vi "Close Module.vi"(7 "Self":refnum<class "UniqueName.lvclass">, 8 "error in (no error)":errorcluster, 9 "Wait for stop?":bool, 11 "Module Admin in":refnum<class "Delacor_lib_QMH_Cloneable Module Admin.lvclass">) -> (0 "error out":errorcluster, 1 "External Launch":bool, 3 "Module Admin out":refnum<class "Delacor_lib_QMH_Cloneable Module Admin.lvclass">)   [LabVIEW 2014, in "Configurable.lvlib"]
doc: "Destroy the Broadcast Events and Request Events (if this was the first instance). Reset flags stored in Module Admin class.\n_____\nBased on Delacor QMH Project Template 4.0.0.47."
uses:
  Configurable.lvlib
  <vilib>/Delacor/Delacor QMH/Libraries/Cloneable Module Admin_class/Delacor_lib_QMH_Cloneable Module Admin.lvclass
  <vilib>/LabVIEW Open Source Project/Unicity/UniqueName/UniqueNameClass/UniqueName.lvclass
  <vilib>/Delacor/Delacor QMH/Libraries/Cloneable Module Admin_class/Delacor_lib_QMH_Cloneable Module Admin.lvclass/Delacor_lib_QMH_Cloneable Module Admin.ctl
  <vilib>/Delacor/Delacor QMH/Libraries/Module Admin_class/Delacor_lib_QMH_Module Admin.lvclass/Delacor_lib_QMH_Module Admin.ctl
  <vilib>/Delacor/Delacor QMH/Libraries/Cloneable Module Admin_class/Delacor_lib_QMH_Get First.vi
  <vilib>/Delacor/Delacor QMH/Libraries/Cloneable Module Admin_class/Delacor_lib_QMH_Get Module ID.vi
  <vilib>/Delacor/Delacor QMH/Libraries/Module Admin_class/Delacor_lib_QMH_Get External Launch.vi
  Clone Registration/Clone Registration.lvlib
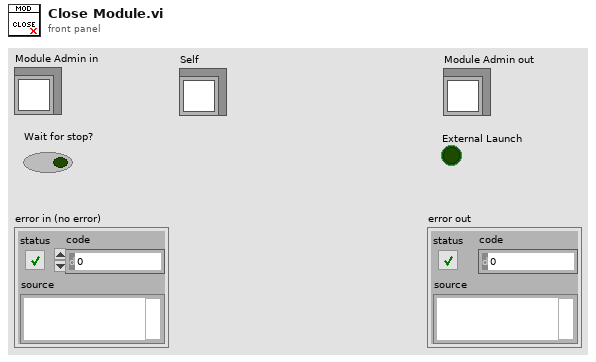
[diagram p1: front panel]
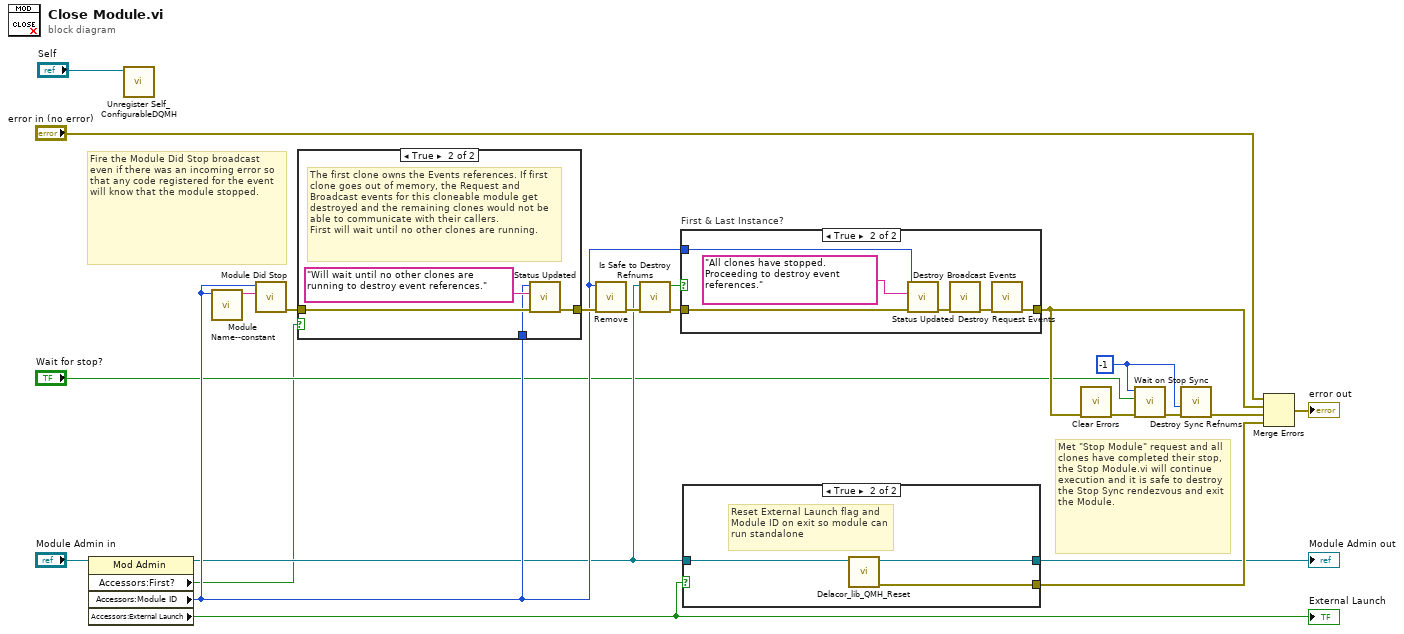
[diagram p0: block diagram]
diagram:
  w8 = -1 ("Module ID")
  # "Fire the Module Did Stop broadcast even if there was an incoming error so that any code registered for the event will know that the module stopped."
  # "Met \"Stop Module\" request and all clones have completed their stop, the Stop Module.vi will continue execution and it is safe to destroy the Stop Sync rendezvous and exit the Module."
  n1 = property class="Mod Admin"(reference="Module Admin in") -> (reference out=w17:refnum<class "Delacor_lib_QMH_Cloneable Module Admin.lvclass">, "Accessors:First?"=w5:bool, "Accessors:Module ID"=w21:i32, "Accessors:External Launch"=w4:bool)  [unwired: 1 in, 1 out]
  "External Launch" <- w4
  n2 = call "Unregister Self_ConfigurableDQMH.vi"("Self"="Self") -> ()  [unwired: 11 in]
  n3 = call "Module Name--constant.vi"("Module ID"=w21) -> ("Module Name"=w3:string)  [unwired: 10 in]
  n4 = call "Module Did Stop.vi"("Origin"=w3, "Module ID"=w21) -> ("error out"=w12:errorcluster)  [unwired: 9 in]
  n5 = case shown="True" w5 {
    tunnel: w12 -> [w23 w27]
    tunnel: w21 -> [_ w25]
    tunnel: [w23 w24] -> w22
    frame False {
    }
    frame True {
      # "The first clone owns the Events references. If first clone goes out of memory, the Request and Broadcast events for this cloneable module get destroyed and the remaining clones would not be able to communicate with their callers.\nFirst will wait until no other clones are running."
      n6 = call "Status Updated.vi"("error in (no error)"=w27, "Status"="Will wait until no other clones are running to destroy event references." ("format string"), "Module ID"=w25) -> ("error out"=w24:errorcluster)  [unwired: 8 in]
    }
  }
  n7 = call "Remove.vi"("error in (no error)"=w22, "Module ID"=w21) -> ("error out"=w18:errorcluster)  [unwired: 8 in, 1 out]
  n8 = call "Is Safe to Destroy Refnums.vi"("error in (no error)"=w18, "Module Admin"=w17) -> ("error out"=w14:errorcluster, "Destroy Broadcast & Request Event Refs?"=w15:bool)  [unwired: 8 in]
  n9 = case "First & Last Instance?" shown="True" w15 {
    tunnel: w14 -> [w28 w32]
    tunnel: [w28 w34] -> w20
    tunnel: w21 -> [_ w30]
    frame False {
    }
    frame True {
      n10 = call "Status Updated.vi"("error in (no error)"=w32, "Status"="All clones have stopped. Proceeding to destroy event references.", "Module ID"=w30) -> ("error out"=w31:errorcluster)  [unwired: 8 in]
      n11 = call "Destroy Broadcast Events.vi"("error in (no error)"=w31) -> ("error out"=w33:errorcluster)  [unwired: 10 in]
      n12 = call "Destroy Request Events.vi"("error in (no error)"=w33) -> ("error out"=w34:errorcluster)  [unwired: 10 in]
    }
  }
  n13 = case shown="True" w4 {
    tunnel: w17 -> [w35 w38]
    tunnel: [w35 w37] -> w13
    tunnel: [_ w36] -> w19
    frame False {
    }
    frame True {
      # "Reset External Launch flag and Module ID on exit so module can run standalone"
      n14 = call-dynamic "Delacor_lib_QMH_Reset.vi"("Mod Admin in"=w38) -> ("error out"=w36:errorcluster, "Mod Admin out"=w37:refnum<class "Delacor_lib_QMH_Cloneable Module Admin.lvclass">)  [unwired: 9 in]
    }
  }
  "Module Admin out" <- w13
  n15 = call <vilib>:"Clear Errors.vi"("error in (no error)"=w20) -> ("error out"=w7:errorcluster)  [unwired: 5 in, 1 out]
  n16 = call "Wait on Stop Sync.vi"("error in (no error)"=w7, "Wait for Module to stop?"="Wait for stop?", "Module ID"=w8) -> ("error out"=w11:errorcluster)  [unwired: 8 in]
  n17 = call "Destroy Sync Refnums.vi"("error in (no error)"=w11, "Module ID"=w8) -> ("error out"=w9:errorcluster)  [unwired: 9 in]
  n18 = Merge Errors("error in (no error)", w20, w9, w19) -> (→"error out":errorcluster)
